vi "FilePathCreation_DCPower_V2.vi"(0 "binary file input reference array 1":refnum<file>[](array[refnum]), 2 "Channel Name Input array":string[](array[string]), 5 "data output directory folder":path, 7 "binary file indexor in":i32, 9 "Reset counter in":i32, 11 "error in (no error)":errorcluster, 12 "binary file input reference array 2":refnum<file>[](array[refnum]), 13 "reset threshold":i32=1000) -> (4 "binary file output reference array":refnum<file>[](array[refnum]), 6 "binary file output reference array 2":refnum<file>[](array[refnum]), 8 "binary file indexor out":i32, 10 "reset counter out":i32, 15 "error out":errorcluster)   [LabVIEW 2019]
panel:
  in  "binary file input reference":refnum<file>
  out "binary file output reference":refnum<file>
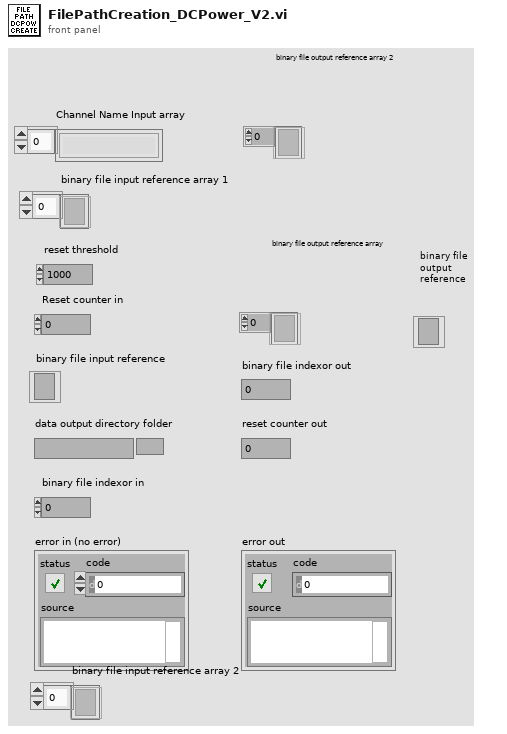
[diagram p1: front panel]
types:
  T1 = enum16{"open", "replace", "create", "open or create", "replace or create", "replace or create with confirmation"}
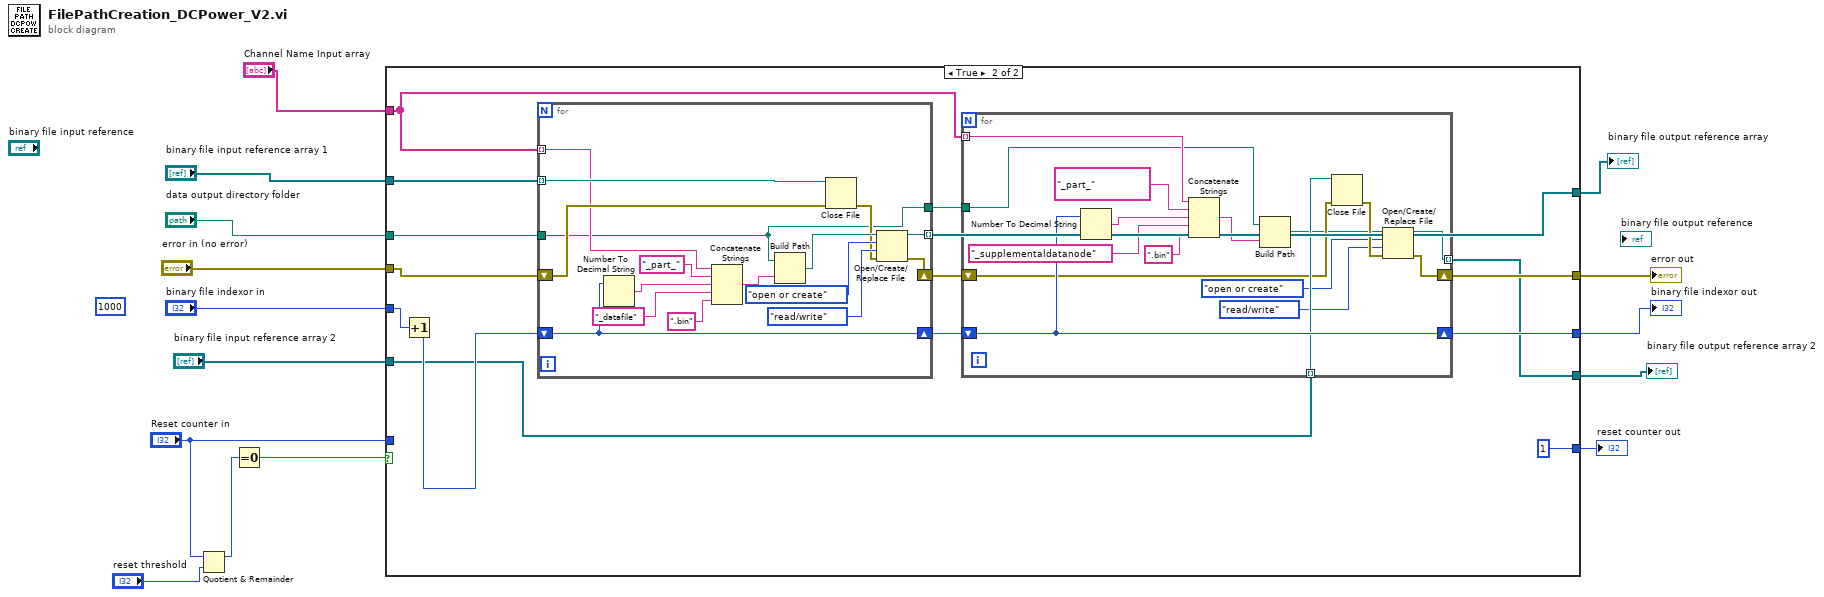
[diagram p0: block diagram]
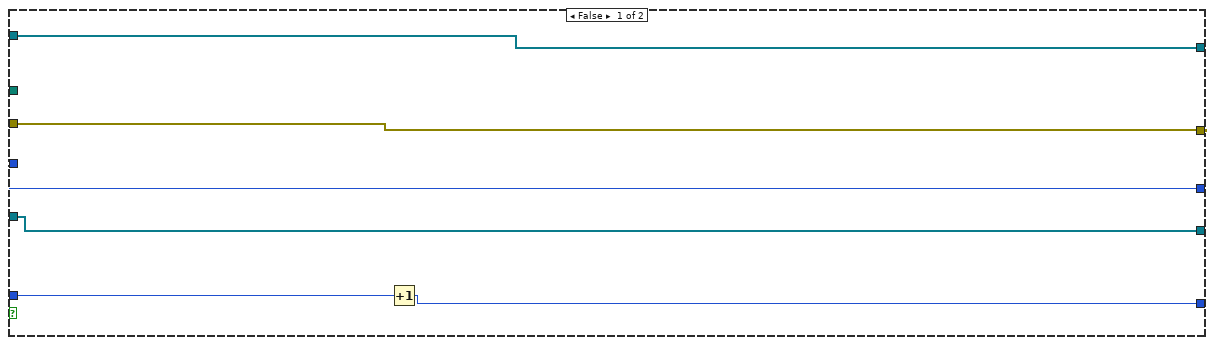
[diagram p2: hidden frame]
diagram:
  (unwired) 1000 ("y")
  n1 = Quotient & Remainder(x="Reset counter in", y="reset threshold") -> (x-y*floor(x/y)=w8:i32)  [unwired: 1 out]
  n2 = Equal To 0?(x=w8) -> (x = 0?=w7:bool)
  n3 = case shown="True" w7 {
    tunnel: [w20 1] -> w13
    tunnel: "Reset counter in" -> [w21 _]
    tunnel: "binary file indexor in" -> [w17 w31]
    tunnel: "binary file input reference array 1" -> [w19 w35]
    tunnel: "error in (no error)" -> [w18 w34]
    tunnel: [w18 w26] -> w11
    tunnel: [w19 w32] -> w3
    tunnel: [w17 w27] -> w12
    tunnel: "data output directory folder" -> [_ w33]
    tunnel: "Channel Name Input array" -> [_ w29]
    tunnel: "binary file input reference array 2" -> [w16 w23]
    tunnel: [w16 w22] -> w1
    frame False {
      n4 = Increment(x=w21) -> (x+1=w20:i32)
    }
    frame True {
      n5 = Increment(x=w31) -> (x+1=w30:i32)
      n6 = for {
        tunnel: w35 -> [w67] mode=indexing
        tunnel: w33 -> [w55]
        tunnel: [w61] -> w32 mode=indexing
        shift-right: [w56] -> w28
        shift-left: w30 -> [w56]
        shift-right: [w60] -> w25
        shift-left: w34 -> [w63]
        tunnel: w29 -> [w57] mode=indexing
        tunnel: [w55] -> w24
        n7 = Number To Decimal String(number=w56) -> (decimal integer string=w59:string)  [unwired: 1 in]
        n8 = Concatenate Strings(w57, "_part_" ("string"), w59, "_datafile" ("string"), ".bin" ("string")) -> (w68:string)
        n9 = Build Path(base path=w55, name or relative path=w68) -> (appended path=w66:path)
        n10 = Close File(refnum=w67, error in=w63) -> (error out=w62:errorcluster)  [unwired: 1 out]
        n11 = Open/Create/Replace File(file path (use dialog)=w66, error in=w62, operation (0:open)=T1."open or create", access (0:read/write)=enum16{"read/write", "read-only", "write-only"}."read/write") -> (refnum out=w61:refnum<file>, error out=w60:errorcluster)  [unwired: 2 in, 1 out]
      }
      n12 = for {
        tunnel: w29 -> [w49] mode=indexing
        shift-right: [w50] -> w27
        shift-left: w28 -> [w50]
        shift-right: [w43] -> w26
        shift-left: w25 -> [w45]
        tunnel: w24 -> [w47]
        tunnel: w23 -> [w46] mode=indexing
        tunnel: [w39] -> w22 mode=indexing
        n13 = Number To Decimal String(number=w50) -> (decimal integer string=w52:string)  [unwired: 1 in]
        n14 = Concatenate Strings(w49, "_part_" ("string"), w52, "_supplementaldatanode" ("string"), ".bin" ("string")) -> (w48:string)
        n15 = Build Path(base path=w47, name or relative path=w48) -> (appended path=w42:path)
        n16 = Close File(refnum=w46, error in=w45) -> (error out=w44:errorcluster)  [unwired: 1 out]
        n17 = Open/Create/Replace File(file path (use dialog)=w42, error in=w44, operation (0:open)=T1."open or create", access (0:read/write)=enum16{"read/write", "read-only", "write-only"}."read/write") -> (refnum out=w39:refnum<file>, error out=w43:errorcluster)  [unwired: 2 in, 1 out]
      }
    }
  }
  "reset counter out" <- w13
  "binary file indexor out" <- w12
  "error out" <- w11
  "binary file output reference array" <- w3
  "binary file output reference array 2" <- w1
